vi "ESP301.vi"() -> ()   [LabVIEW 2014]
uses:
  ESP301/Newport ESP301.lvlib
panel:
  in  "stop":bool
  in  "AxisNumTiltY":dbl
  in  "AxisNumTiltX":dbl
  in  "AxisNumZ":dbl
  in  "AxisNumY":dbl
  in  "AxisNumX":dbl
  in  "Tilt  Y":T1 {"Actual Velocity" min=0.0 max=12.7 format="%1.5g"; "Move Relative" min=0.0 max=12.0 format="%1.5f"; "Set Velocity" min=0.0 max=0.2 format="%1.4f"; "Actual Position" format="%1.6f"; "Move Absolute" min=0.0 max=12.7 format="%1.5f"}
  in  "Tilt  X":T1 {"Actual Velocity" min=0.0 max=12.7 format="%1.5g"; "Move Relative" min=0.0 max=12.0 format="%1.5f"; "Set Velocity" min=0.0 max=0.2 format="%1.4f"; "Actual Position" format="%1.6f"; "Move Absolute" min=0.0 max=12.7 format="%1.5f"}
  in  "Axis Z":T1 {"Actual Velocity" min=0.0 max=12.7 format="%1.5g"; "Move Relative" min=0.0 max=12.0 format="%1.5f"; "Set Velocity" min=0.0 max=0.2 format="%1.4f"; "Actual Position" format="%1.6f"; "Move Absolute" min=0.0 max=12.7 format="%1.5f"}
  in  "Axis Y":T1 {"Actual Velocity" min=0.0 max=12.7 format="%1.5g"; "Move Relative" min=0.0 max=12.0 format="%1.5f"; "Set Velocity" min=0.0 max=0.2 format="%1.4f"; "Actual Position" format="%1.6f"; "Move Absolute" min=0.0 max=12.7 format="%1.5f"}
  in  "Axis X":T1 {"Actual Velocity" min=0.0 max=12.7 format="%1.5g"; "Move Relative" min=0.0 max=12.0 format="%1.5f"; "Set Velocity" min=0.0 max=0.2 format="%1.4f"; "Actual Position" format="%1.6f"; "Move Absolute" min=0.0 max=12.7 format="%1.5f"}
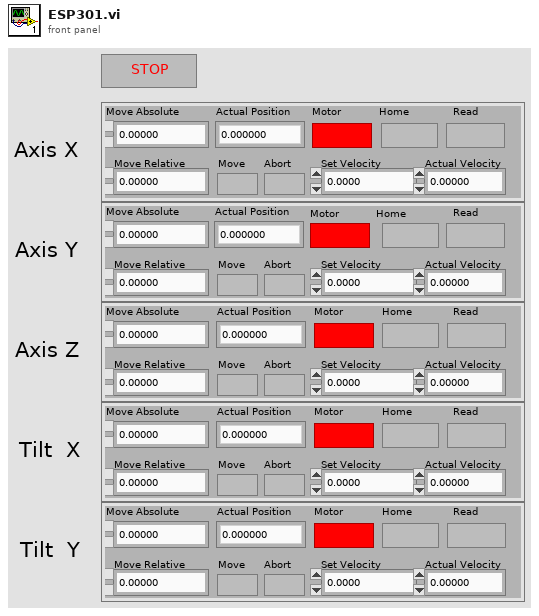
[diagram p1: front panel]
types:
  T1 = cluster{"Move Absolute":dbl, "Actual Position":dbl, "Motor":bool, "Home":bool, "Set Velocity":dbl, "Move Relative":dbl, "Actual Velocity":dbl, "Move":bool, "Read":bool, "Abort":bool}
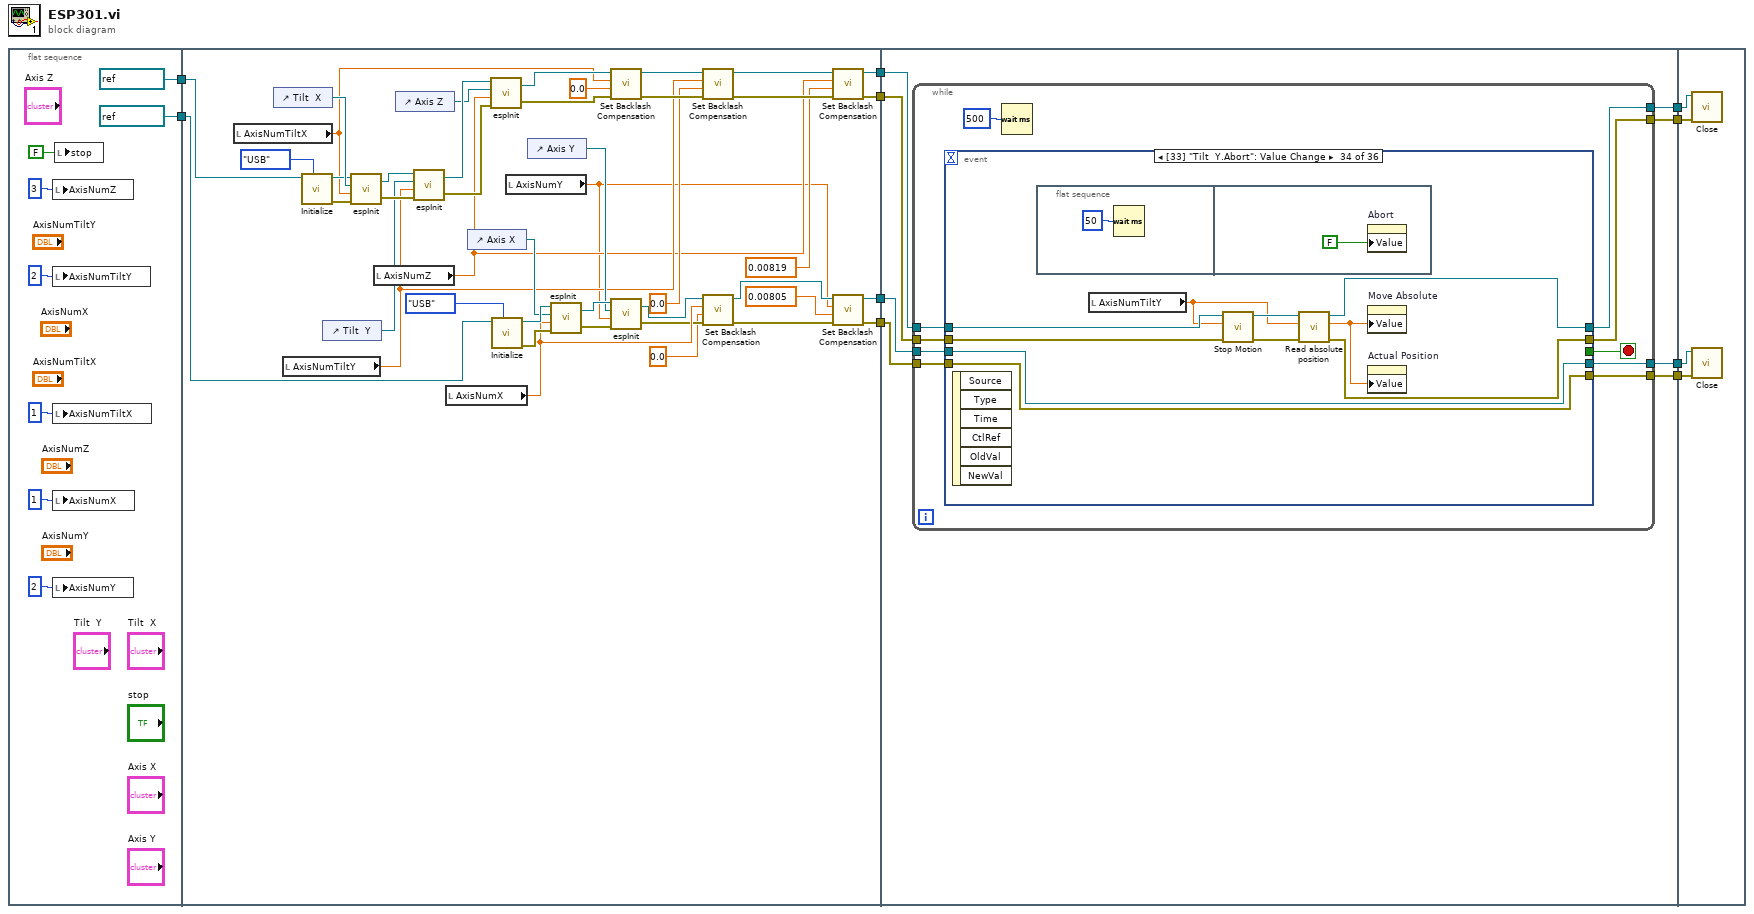
[diagram p0: block diagram]
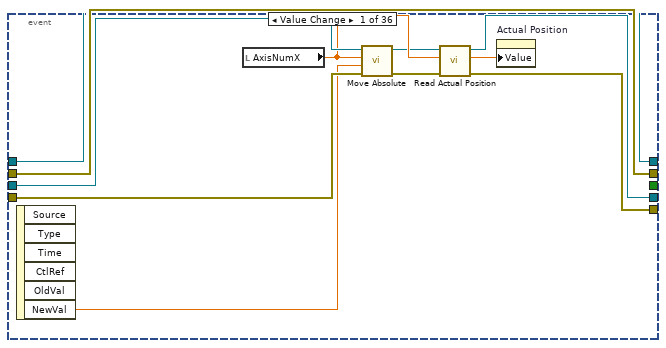
[diagram p2: hidden frame]
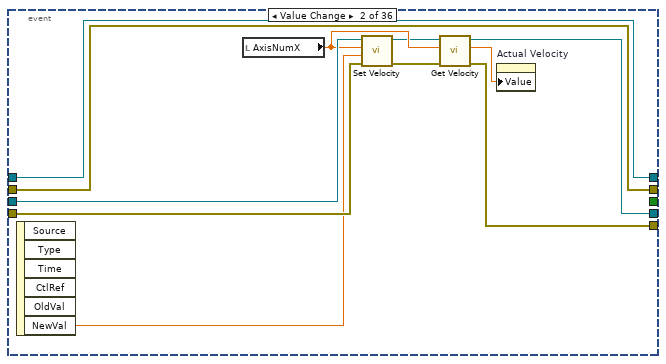
[diagram p3: hidden frame]
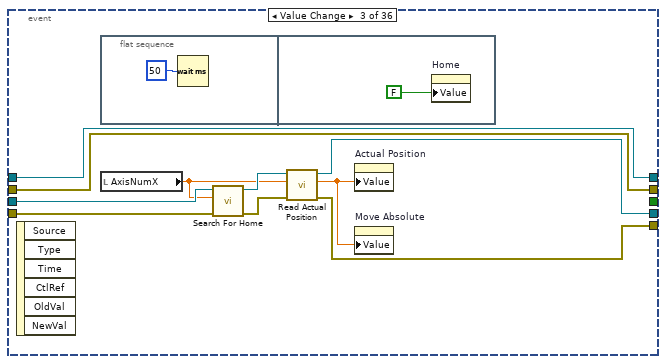
[diagram p4: hidden frame]
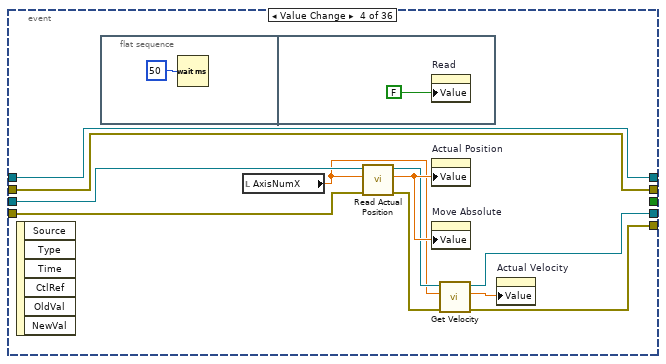
[diagram p5: hidden frame]
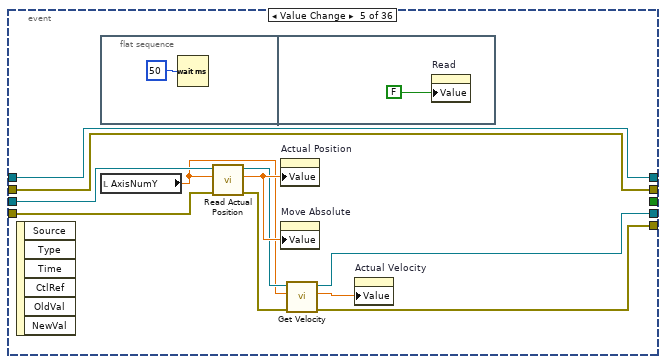
[diagram p6: hidden frame]
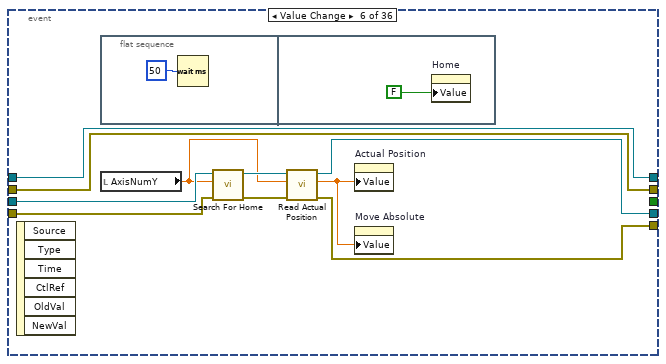
[diagram p7: hidden frame]
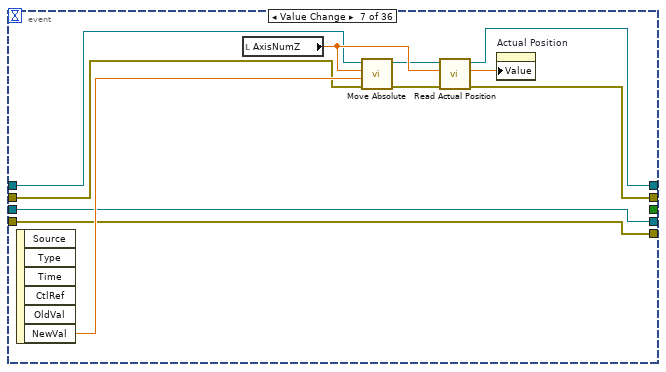
[diagram p8: hidden frame]
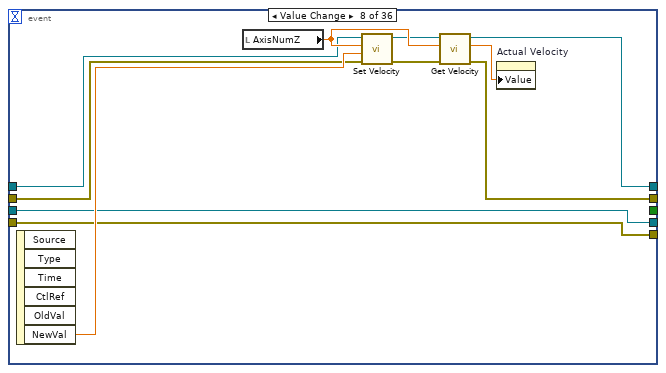
[diagram p9: hidden frame]
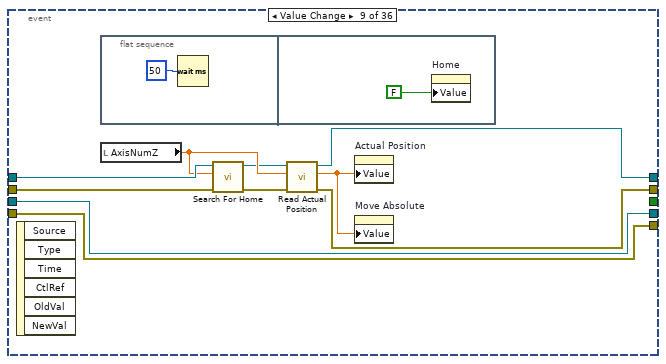
[diagram p10: hidden frame]
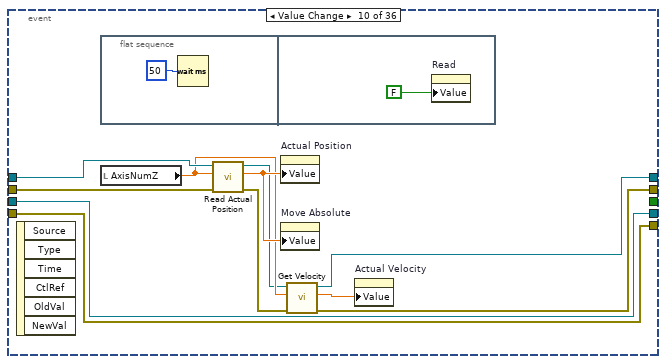
[diagram p11: hidden frame]
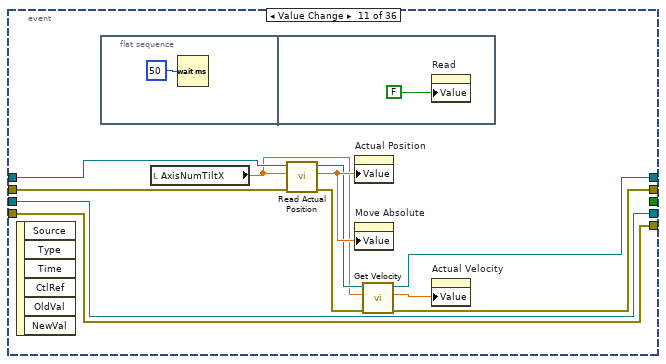
[diagram p12: hidden frame]
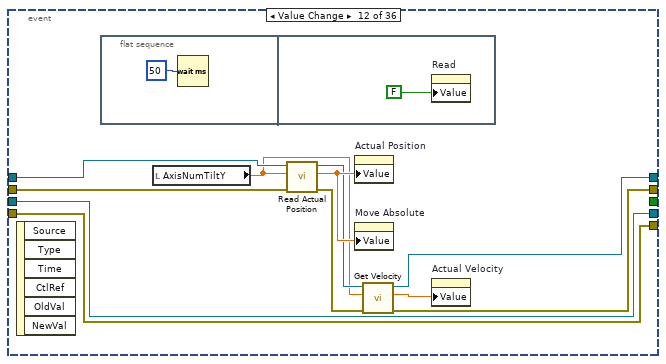
[diagram p13: hidden frame]
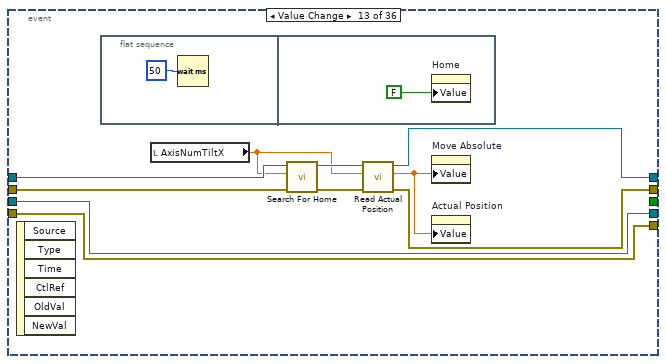
[diagram p14: hidden frame]
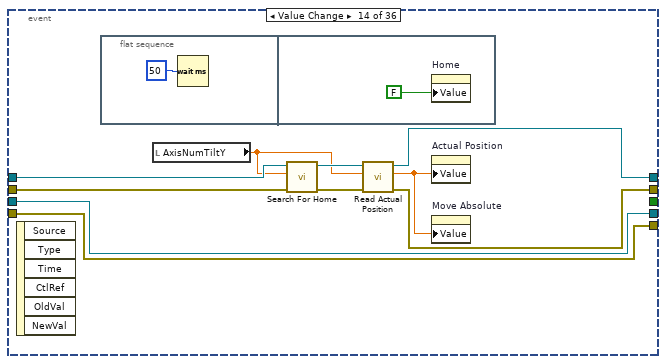
[diagram p15: hidden frame]
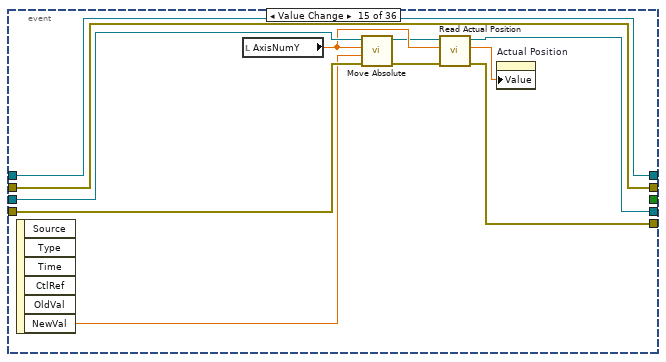
[diagram p16: hidden frame]
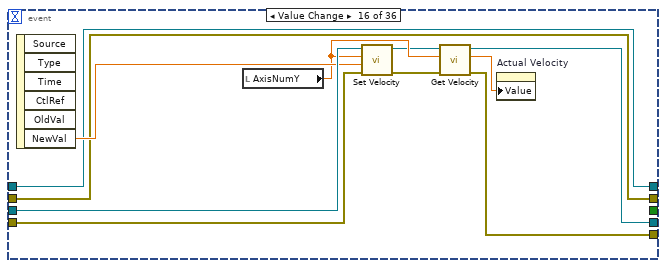
[diagram p17: hidden frame]
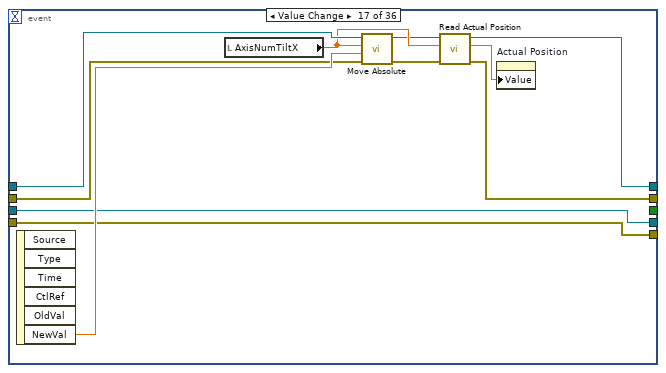
[diagram p18: hidden frame]
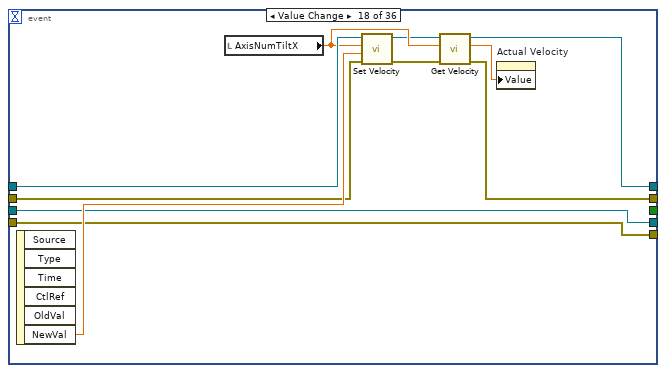
[diagram p19: hidden frame]
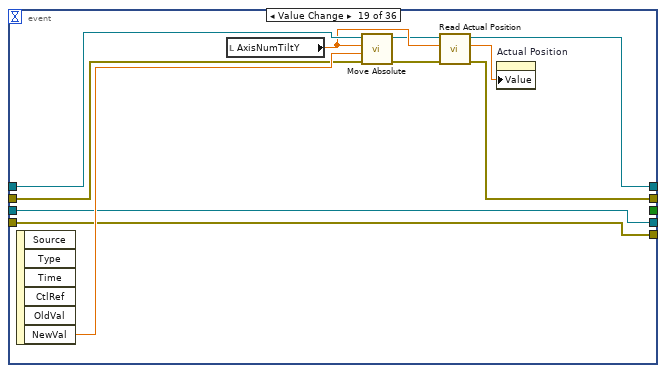
[diagram p20: hidden frame]
diagram:
  n1 = flat-sequence {
    tunnel: [refnum<visa-resource-name> "COM4" ("VISA resource name")] -> w7
    tunnel: [refnum<visa-resource-name> "COM5" ("VISA resource name")] -> w6
    tunnel: [w23] -> w10
    tunnel: [w30] -> w9
    tunnel: [w29] -> w8
    tunnel: w7 -> [w44]
    tunnel: w6 -> [w43]
    tunnel: [w24] -> w5
    tunnel: w10 -> [w68]
    tunnel: w9 -> [w67]
    tunnel: w8 -> [w66]
    tunnel: w5 -> [w69]
    tunnel: [w65] -> w4
    tunnel: [w64] -> w3
    tunnel: [w63] -> w2
    tunnel: [w62] -> w1
    tunnel: w4 -> [w489]
    tunnel: w3 -> [w492]
    tunnel: w2 -> [w491]
    tunnel: w1 -> [w490]
    frame #0 {
      n2 = local write "AxisNumZ"(3) -> ()
      n3 = local write "AxisNumTiltY"(2) -> ()
      n4 = local write "AxisNumTiltX"(1) -> ()
      n5 = local write "AxisNumX"(1 ("AxisNumX")) -> ()
      n6 = local write "AxisNumY"(2) -> ()
      n7 = local write "stop"(FALSE) -> ()
    }
    frame #1 {
      n8 = local read "AxisNumTiltX"() -> (w39:dbl)
      n9 = control-ref of="Tilt  X"() -> (w50:refnum<vi>)
      n10 = local read "AxisNumTiltY"() -> (w36:dbl)
      n11 = call <instrlib>:"Initialize.vi"("VISA resource name"=w44, "Serial Link (RS232)"=enum16{"RS232", "USB"}."USB") -> ("VISA resource name out"=w49:refnum<visa-resource-name>, "error out"=w58:errorcluster)  [unwired: 7 in]
      n12 = control-ref of="Tilt  Y"() -> (w47:refnum<vi>)
      n13 = call "espInit.vi"("error in (no error)"=w58, "Axis"=w39, "RefNum"=w50, "VISA resource name in"=w49) -> ("error out"=w56:errorcluster, "VISA resource name out"=w57:refnum<visa-resource-name>)
      n14 = local read "AxisNumZ"() -> (w32:dbl)
      n15 = control-ref of="Axis Z"() -> (w48:refnum<vi>)
      n16 = call "espInit.vi"("error in (no error)"=w56, "Axis"=w36, "RefNum"=w47, "VISA resource name in"=w57) -> ("error out"=w54:errorcluster, "VISA resource name out"=w55:refnum<visa-resource-name>)
      n17 = local read "AxisNumX"() -> (w26:dbl)
      n18 = control-ref of="Axis X"() -> (w46:refnum<vi>)
      n19 = call "espInit.vi"("error in (no error)"=w54, "Axis"=w32, "RefNum"=w48, "VISA resource name in"=w55) -> ("error out"=w41:errorcluster, "VISA resource name out"=w42:refnum<visa-resource-name>)
      n20 = call <instrlib>:"Initialize.vi"("VISA resource name"=w43, "Serial Link (RS232)"=enum16{"RS232", "USB"}."USB") -> ("VISA resource name out"=w52:refnum<visa-resource-name>, "error out"=w51:errorcluster)  [unwired: 7 in]
      n21 = local read "AxisNumY"() -> (w25:dbl)
      n22 = control-ref of="Axis Y"() -> (w45:refnum<vi>)
      n23 = call "espInit.vi"("error in (no error)"=w51, "Axis"=w26, "RefNum"=w46, "VISA resource name in"=w52) -> ("error out"=w60:errorcluster, "VISA resource name out"=w61:refnum<visa-resource-name>)
      n24 = call <instrlib>:"Set Backlash Compensation.vi"("error in (no error)"=w41, "Backlash Compensation Value (0 units)"=0.0, "Axis (1)"=w39, "VISA resource name"=w42) -> ("error out"=w37:errorcluster, "VISA resource name out"=w38:refnum<visa-resource-name>)  [unwired: 2 in]
      n25 = call "espInit.vi"("error in (no error)"=w60, "Axis"=w25, "RefNum"=w45, "VISA resource name in"=w61) -> ("error out"=w21:errorcluster, "VISA resource name out"=w22:refnum<visa-resource-name>)
      n26 = call <instrlib>:"Set Backlash Compensation.vi"("error in (no error)"=w37, "Backlash Compensation Value (0 units)"=0.0, "Axis (1)"=w36, "VISA resource name"=w38) -> ("error out"=w33:errorcluster, "VISA resource name out"=w34:refnum<visa-resource-name>)  [unwired: 2 in]
      n27 = call <instrlib>:"Set Backlash Compensation.vi"("error in (no error)"=w21, "Backlash Compensation Value (0 units)"=0.0, "Axis (1)"=w26, "VISA resource name"=w22) -> ("error out"=w27:errorcluster, "VISA resource name out"=w28:refnum<visa-resource-name>)  [unwired: 2 in]
      n28 = call <instrlib>:"Set Backlash Compensation.vi"("error in (no error)"=w33, "Backlash Compensation Value (0 units)"=0.00819, "Axis (1)"=w32, "VISA resource name"=w34) -> ("error out"=w29:errorcluster, "VISA resource name out"=w30:refnum<visa-resource-name>)  [unwired: 2 in]
      n29 = call <instrlib>:"Set Backlash Compensation.vi"("error in (no error)"=w27, "Backlash Compensation Value (0 units)"=0.00805, "Axis (1)"=w25, "VISA resource name"=w28) -> ("error out"=w23:errorcluster, "VISA resource name out"=w24:refnum<visa-resource-name>)  [unwired: 2 in]
    }
    frame #2 {
      n30 = while {
        tunnel: w67 -> [w79]
        tunnel: w66 -> [w78]
        tunnel: w69 -> [w77]
        tunnel: w68 -> [w76]
        tunnel: [w75] -> w65
        tunnel: [w74] -> w64
        tunnel: [w73] -> w63
        tunnel: [w72] -> w62
        stop <- w70 stop-if-true
        n31 = event shown="[33] \"Tilt  Y.Abort\": Value Change" {
          selector: _ -> [_ _ _ _ _ _ _ _ _ _ _ _ _ _ _ _ _ _ _ _ _ _ _ _ _ _ _ _ _ _ _ _ _ _ _ _]
          dyn-events: _ -> [_ _ _ _ _ _ _ _ _ _ _ _ _ _ _ _ _ _ _ _ _ _ _ _ _ _ _ _ _ _ _ _ _ _ _ _]
          timeout: _ -> [_ _ _ _ _ _ _ _ _ _ _ _ _ _ _ _ _ _ _ _ _ _ _ _ _ _ _ _ _ _ _ _ _ _ _ _]
          tunnel: w79 -> [w81 w92 w103 w121 w134 w141 w157 w168 w183 w195 w209 w222 w234 w246 w252 w263 w279 w290 w301 w312 w316 w330 w340 w347 w359 w363 w375 w383 w387 w405 w419 w433 w451 w463 _ w478]
          tunnel: w78 -> [w80 w91 w102 w120 w133 w140 w156 w167 w182 w194 w208 w221 w233 w245 w251 w262 w278 w289 w300 w311 w315 w329 w341 w346 w358 w362 w374 w382 w386 w404 w418 w432 w450 w462 w466 w477]
          tunnel: w77 -> [w90 w101 w111 w124 w137 w149 w153 w164 w175 w193 w206 w219 w225 w238 w259 w270 w274 w285 w296 w307 w325 w334 w339 w344 w351 w367 w370 w381 w396 w401 w414 w429 w443 w455 w470 w482]
          tunnel: w76 -> [w89 w100 w110 w123 w136 w148 w152 w163 w174 w192 w205 w218 w226 w237 w258 w269 w273 w284 w295 w306 w324 w333 w338 w342 w350 w366 w373 w380 w395 w400 w415 w428 w442 w454 w469 w481]
          tunnel: [w87 w98 w107 w116 w130 w143 w153 w164 w175 w193 w206 w219 w225 w238 w255 w266 w274 w285 w296 w307 w320 w332 w339 w344 w351 w365 w370 w381 w391 w401 w414 w429 w443 w455 w468 w480] -> w73
          tunnel: [w86 w97 w106 w115 w129 w147 w152 w163 w174 w192 w205 w218 w226 w237 w254 w265 w273 w284 w295 w306 w319 w331 w338 w342 w350 w364 w373 w380 w390 w400 w415 w428 w442 w454 w467 w479] -> w72
          tunnel: [w81 w92 w103 w121 w134 w141 w160 w171 w181 w187 w199 w214 w232 w242 w252 w263 w276 w287 w298 w309 w316 w330 w340 w345 w355 w363 w371 w379 w387 w402 w416 w430 w447 w459 _ w478] -> w75
          tunnel: [w80 w91 w102 w120 w133 w140 w159 w170 w180 w186 w200 w213 w231 w241 w251 w262 w275 w286 w297 w308 w315 w329 w341 w343 w354 w362 w372 w378 w386 w403 w417 w431 w446 w458 w466 w477] -> w74
          tunnel: [_ _ _ _ _ _ _ _ _ _ _ _ _ _ _ _ _ _ _ _ _ _ w337 _ _ _ _ _ _ _ _ _ _ _ _ _] -> w70
          event "Axis X.Move Absolute": Value Change {
            n32 = event-data() -> ("NewVal"=w88:dbl)  [unwired: 1 in, 5 out]
            n33 = local read "AxisNumX"() -> (w84:dbl)
            n34 = call <instrlib>:"Move Absolute.vi"("error in (no error)"=w89, "Position (0 units)"=w88, "Axis (1)"=w84, "VISA resource name"=w90) -> ("error out"=w82:errorcluster, "VISA resource name out"=w83:refnum<visa-resource-name>)  [unwired: 2 in]
            n35 = call <instrlib>:"Read Actual Position.vi"("error in (no error)"=w82, "Axis (1)"=w84, "VISA resource name"=w83) -> ("error out"=w86:errorcluster, "Position (units)"=w85:dbl, "VISA resource name out"=w87:refnum<visa-resource-name>)  [unwired: 2 in]
            n36 = property on="Actual Position" class="DigNum (strict)"("Value"=w85) -> ()  [unwired: 2 in, 2 out]
          }
          event "Axis X.Set Velocity": Value Change {
            n37 = event-data() -> ("NewVal"=w99:dbl)  [unwired: 1 in, 5 out]
            n38 = local read "AxisNumX"() -> (w95:dbl)
            n39 = call <instrlib>:"Set Velocity.vi"("error in (no error)"=w100, "Velocity (units/s)"=w99, "Axis (1)"=w95, "VISA resource name"=w101) -> ("error out"=w93:errorcluster, "VISA resource name out"=w94:refnum<visa-resource-name>)  [unwired: 2 in]
            n40 = call "Get Velocity.vi"("error in (no error)"=w93, "Axis (1)"=w95, "VISA resource name"=w94) -> ("error out"=w97:errorcluster, "Velocity (units/s)"=w96:dbl, "VISA resource name out"=w98:refnum<visa-resource-name>)  [unwired: 2 in]
            n41 = property on="Actual Velocity" class="DigNum (strict)"("Value"=w96) -> ()  [unwired: 2 in, 2 out]
          }
          event "Axis X.Home": Value Change {
            n42 = event-data() -> ()  [unwired: 1 in, 6 out]
            n43 = flat-sequence {
              frame #0 {
                n44 = Wait (ms)(milliseconds to wait=u32 50) -> ()  [unwired: 1 out]
              }
              frame #1 {
                n45 = property on="Home" class="Bool (strict)"("Value"=FALSE) -> ()  [unwired: 2 in, 2 out]
              }
            }
            n46 = local read "AxisNumX"() -> (w105:dbl)
            n47 = call <instrlib>:"Search For Home.vi"("error in (no error)"=w110, "Axis (1)"=w105, "VISA resource name"=w111) -> ("error out"=w108:errorcluster, "VISA resource name out"=w109:refnum<visa-resource-name>)  [unwired: 4 in]
            n48 = call <instrlib>:"Read Actual Position.vi"("error in (no error)"=w108, "Axis (1)"=w105, "VISA resource name"=w109) -> ("error out"=w106:errorcluster, "Position (units)"=w104:dbl, "VISA resource name out"=w107:refnum<visa-resource-name>)  [unwired: 2 in]
            n49 = property on="Actual Position" class="DigNum (strict)"("Value"=w104) -> ()  [unwired: 2 in, 2 out]
            n50 = property on="Move Absolute" class="DigNum (strict)"("Value"=w104) -> ()  [unwired: 2 in, 2 out]
          }
          event "Axis X.Read": Value Change {
            n51 = event-data() -> ()  [unwired: 1 in, 6 out]
            n52 = flat-sequence {
              frame #0 {
                n53 = Wait (ms)(milliseconds to wait=u32 50) -> ()  [unwired: 1 out]
              }
              frame #1 {
                n54 = property on="Read" class="Bool (strict)"("Value"=FALSE) -> ()  [unwired: 2 in, 2 out]
              }
            }
            n55 = local read "AxisNumX"() -> (w117:dbl)
            n56 = call <instrlib>:"Read Actual Position.vi"("error in (no error)"=w123, "Axis (1)"=w117, "VISA resource name"=w124) -> ("error out"=w118:errorcluster, "Position (units)"=w122:dbl, "VISA resource name out"=w119:refnum<visa-resource-name>)  [unwired: 2 in]
            n57 = property on="Actual Position" class="DigNum (strict)"("Value"=w122) -> ()  [unwired: 2 in, 2 out]
            n58 = property on="Move Absolute" class="DigNum (strict)"("Value"=w122) -> ()  [unwired: 2 in, 2 out]
            n59 = call "Get Velocity.vi"("error in (no error)"=w118, "Axis (1)"=w117, "VISA resource name"=w119) -> ("error out"=w115:errorcluster, "Velocity (units/s)"=w114:dbl, "VISA resource name out"=w116:refnum<visa-resource-name>)  [unwired: 2 in]
            n60 = property on="Actual Velocity" class="DigNum (strict)"("Value"=w114) -> ()  [unwired: 2 in, 2 out]
          }
          event "Axis Y.Read": Value Change {
            n61 = event-data() -> ()  [unwired: 1 in, 6 out]
            n62 = flat-sequence {
              frame #0 {
                n63 = Wait (ms)(milliseconds to wait=u32 50) -> ()  [unwired: 1 out]
              }
              frame #1 {
                n64 = property on="Read" class="Bool (strict)"("Value"=FALSE) -> ()  [unwired: 2 in, 2 out]
              }
            }
            n65 = local read "AxisNumY"() -> (w128:dbl)
            n66 = call <instrlib>:"Read Actual Position.vi"("error in (no error)"=w136, "Axis (1)"=w128, "VISA resource name"=w137) -> ("error out"=w131:errorcluster, "Position (units)"=w135:dbl, "VISA resource name out"=w132:refnum<visa-resource-name>)  [unwired: 2 in]
            n67 = property on="Actual Position" class="DigNum (strict)"("Value"=w135) -> ()  [unwired: 2 in, 2 out]
            n68 = property on="Move Absolute" class="DigNum (strict)"("Value"=w135) -> ()  [unwired: 2 in, 2 out]
            n69 = call "Get Velocity.vi"("error in (no error)"=w131, "Axis (1)"=w128, "VISA resource name"=w132) -> ("error out"=w129:errorcluster, "Velocity (units/s)"=w127:dbl, "VISA resource name out"=w130:refnum<visa-resource-name>)  [unwired: 2 in]
            n70 = property on="Actual Velocity" class="DigNum (strict)"("Value"=w127) -> ()  [unwired: 2 in, 2 out]
          }
          event "Axis Y.Home": Value Change {
            n71 = event-data() -> ()  [unwired: 1 in, 6 out]
            n72 = flat-sequence {
              frame #0 {
                n73 = Wait (ms)(milliseconds to wait=u32 50) -> ()  [unwired: 1 out]
              }
              frame #1 {
                n74 = property on="Home" class="Bool (strict)"("Value"=FALSE) -> ()  [unwired: 2 in, 2 out]
              }
            }
            n75 = local read "AxisNumY"() -> (w144:dbl)
            n76 = call <instrlib>:"Search For Home.vi"("error in (no error)"=w148, "Axis (1)"=w144, "VISA resource name"=w149) -> ("error out"=w145:errorcluster, "VISA resource name out"=w146:refnum<visa-resource-name>)  [unwired: 4 in]
            n77 = call <instrlib>:"Read Actual Position.vi"("error in (no error)"=w145, "Axis (1)"=w144, "VISA resource name"=w146) -> ("error out"=w147:errorcluster, "Position (units)"=w142:dbl, "VISA resource name out"=w143:refnum<visa-resource-name>)  [unwired: 2 in]
            n78 = property on="Actual Position" class="DigNum (strict)"("Value"=w142) -> ()  [unwired: 2 in, 2 out]
            n79 = property on="Move Absolute" class="DigNum (strict)"("Value"=w142) -> ()  [unwired: 2 in, 2 out]
          }
          event "Axis Z.Move Absolute": Value Change {
            n80 = event-data() -> ("NewVal"=w162:dbl)  [unwired: 1 in, 5 out]
            n81 = local read "AxisNumZ"() -> (w158:dbl)
            n82 = call <instrlib>:"Move Absolute.vi"("error in (no error)"=w156, "Position (0 units)"=w162, "Axis (1)"=w158, "VISA resource name"=w157) -> ("error out"=w154:errorcluster, "VISA resource name out"=w155:refnum<visa-resource-name>)  [unwired: 2 in]
            n83 = call <instrlib>:"Read Actual Position.vi"("error in (no error)"=w154, "Axis (1)"=w158, "VISA resource name"=w155) -> ("error out"=w159:errorcluster, "Position (units)"=w161:dbl, "VISA resource name out"=w160:refnum<visa-resource-name>)  [unwired: 2 in]
            n84 = property on="Actual Position" class="DigNum (strict)"("Value"=w161) -> ()  [unwired: 2 in, 2 out]
          }
          event "Axis Z.Set Velocity": Value Change {
            n85 = event-data() -> ("NewVal"=w173:dbl)  [unwired: 1 in, 5 out]
            n86 = local read "AxisNumZ"() -> (w169:dbl)
            n87 = call <instrlib>:"Set Velocity.vi"("error in (no error)"=w167, "Velocity (units/s)"=w173, "Axis (1)"=w169, "VISA resource name"=w168) -> ("error out"=w165:errorcluster, "VISA resource name out"=w166:refnum<visa-resource-name>)  [unwired: 2 in]
            n88 = call "Get Velocity.vi"("error in (no error)"=w165, "Axis (1)"=w169, "VISA resource name"=w166) -> ("error out"=w170:errorcluster, "Velocity (units/s)"=w172:dbl, "VISA resource name out"=w171:refnum<visa-resource-name>)  [unwired: 2 in]
            n89 = property on="Actual Velocity" class="DigNum (strict)"("Value"=w172) -> ()  [unwired: 2 in, 2 out]
          }
          event "Axis Z.Home": Value Change {
            n90 = event-data() -> ()  [unwired: 1 in, 6 out]
            n91 = flat-sequence {
              frame #0 {
                n92 = Wait (ms)(milliseconds to wait=u32 50) -> ()  [unwired: 1 out]
              }
              frame #1 {
                n93 = property on="Home" class="Bool (strict)"("Value"=FALSE) -> ()  [unwired: 2 in, 2 out]
              }
            }
            n94 = local read "AxisNumZ"() -> (w179:dbl)
            n95 = call <instrlib>:"Search For Home.vi"("error in (no error)"=w182, "Axis (1)"=w179, "VISA resource name"=w183) -> ("error out"=w178:errorcluster, "VISA resource name out"=w177:refnum<visa-resource-name>)  [unwired: 4 in]
            n96 = call <instrlib>:"Read Actual Position.vi"("error in (no error)"=w178, "Axis (1)"=w179, "VISA resource name"=w177) -> ("error out"=w180:errorcluster, "Position (units)"=w176:dbl, "VISA resource name out"=w181:refnum<visa-resource-name>)  [unwired: 2 in]
            n97 = property on="Actual Position" class="DigNum (strict)"("Value"=w176) -> ()  [unwired: 2 in, 2 out]
            n98 = property on="Move Absolute" class="DigNum (strict)"("Value"=w176) -> ()  [unwired: 2 in, 2 out]
          }
          event "Axis Z.Read": Value Change {
            n99 = event-data() -> ()  [unwired: 1 in, 6 out]
            n100 = flat-sequence {
              frame #0 {
                n101 = Wait (ms)(milliseconds to wait=u32 50) -> ()  [unwired: 1 out]
              }
              frame #1 {
                n102 = property on="Read" class="Bool (strict)"("Value"=FALSE) -> ()  [unwired: 2 in, 2 out]
              }
            }
            n103 = local read "AxisNumZ"() -> (w190:dbl)
            n104 = call <instrlib>:"Read Actual Position.vi"("error in (no error)"=w194, "Axis (1)"=w190, "VISA resource name"=w195) -> ("error out"=w188:errorcluster, "Position (units)"=w196:dbl, "VISA resource name out"=w189:refnum<visa-resource-name>)  [unwired: 2 in]
            n105 = property on="Actual Position" class="DigNum (strict)"("Value"=w196) -> ()  [unwired: 2 in, 2 out]
            n106 = property on="Move Absolute" class="DigNum (strict)"("Value"=w196) -> ()  [unwired: 2 in, 2 out]
            n107 = call "Get Velocity.vi"("error in (no error)"=w188, "Axis (1)"=w190, "VISA resource name"=w189) -> ("error out"=w186:errorcluster, "Velocity (units/s)"=w191:dbl, "VISA resource name out"=w187:refnum<visa-resource-name>)  [unwired: 2 in]
            n108 = property on="Actual Velocity" class="DigNum (strict)"("Value"=w191) -> ()  [unwired: 2 in, 2 out]
          }
          event "Tilt  X.Read": Value Change {
            n109 = event-data() -> ()  [unwired: 1 in, 6 out]
            n110 = flat-sequence {
              frame #0 {
                n111 = Wait (ms)(milliseconds to wait=u32 50) -> ()  [unwired: 1 out]
              }
              frame #1 {
                n112 = property on="Read" class="Bool (strict)"("Value"=FALSE) -> ()  [unwired: 2 in, 2 out]
              }
            }
            n113 = local read "AxisNumTiltX"() -> (w202:dbl)
            n114 = call <instrlib>:"Read Actual Position.vi"("error in (no error)"=w208, "Axis (1)"=w202, "VISA resource name"=w209) -> ("error out"=w201:errorcluster, "Position (units)"=w207:dbl, "VISA resource name out"=w203:refnum<visa-resource-name>)  [unwired: 2 in]
            n115 = property on="Actual Position" class="DigNum (strict)"("Value"=w207) -> ()  [unwired: 2 in, 2 out]
            n116 = property on="Move Absolute" class="DigNum (strict)"("Value"=w207) -> ()  [unwired: 2 in, 2 out]
            n117 = call "Get Velocity.vi"("error in (no error)"=w201, "Axis (1)"=w202, "VISA resource name"=w203) -> ("error out"=w200:errorcluster, "Velocity (units/s)"=w204:dbl, "VISA resource name out"=w199:refnum<visa-resource-name>)  [unwired: 2 in]
            n118 = property on="Actual Velocity" class="DigNum (strict)"("Value"=w204) -> ()  [unwired: 2 in, 2 out]
          }
          event "Tilt  Y.Read": Value Change {
            n119 = event-data() -> ()  [unwired: 1 in, 6 out]
            n120 = flat-sequence {
              frame #0 {
                n121 = Wait (ms)(milliseconds to wait=u32 50) -> ()  [unwired: 1 out]
              }
              frame #1 {
                n122 = property on="Read" class="Bool (strict)"("Value"=FALSE) -> ()  [unwired: 2 in, 2 out]
              }
            }
            n123 = local read "AxisNumTiltY"() -> (w212:dbl)
            n124 = call <instrlib>:"Read Actual Position.vi"("error in (no error)"=w221, "Axis (1)"=w212, "VISA resource name"=w222) -> ("error out"=w215:errorcluster, "Position (units)"=w220:dbl, "VISA resource name out"=w216:refnum<visa-resource-name>)  [unwired: 2 in]
            n125 = property on="Actual Position" class="DigNum (strict)"("Value"=w220) -> ()  [unwired: 2 in, 2 out]
            n126 = property on="Move Absolute" class="DigNum (strict)"("Value"=w220) -> ()  [unwired: 2 in, 2 out]
            n127 = call "Get Velocity.vi"("error in (no error)"=w215, "Axis (1)"=w212, "VISA resource name"=w216) -> ("error out"=w213:errorcluster, "Velocity (units/s)"=w217:dbl, "VISA resource name out"=w214:refnum<visa-resource-name>)  [unwired: 2 in]
            n128 = property on="Actual Velocity" class="DigNum (strict)"("Value"=w217) -> ()  [unwired: 2 in, 2 out]
          }
          event "Tilt  X.Home": Value Change {
            n129 = event-data() -> ()  [unwired: 1 in, 6 out]
            n130 = flat-sequence {
              frame #0 {
                n131 = Wait (ms)(milliseconds to wait=u32 50) -> ()  [unwired: 1 out]
              }
              frame #1 {
                n132 = property on="Home" class="Bool (strict)"("Value"=FALSE) -> ()  [unwired: 2 in, 2 out]
              }
            }
            n133 = local read "AxisNumTiltX"() -> (w228:dbl)
            n134 = call <instrlib>:"Search For Home.vi"("error in (no error)"=w233, "Axis (1)"=w228, "VISA resource name"=w234) -> ("error out"=w230:errorcluster, "VISA resource name out"=w229:refnum<visa-resource-name>)  [unwired: 4 in]
            n135 = call <instrlib>:"Read Actual Position.vi"("error in (no error)"=w230, "Axis (1)"=w228, "VISA resource name"=w229) -> ("error out"=w231:errorcluster, "Position (units)"=w227:dbl, "VISA resource name out"=w232:refnum<visa-resource-name>)  [unwired: 2 in]
            n136 = property on="Move Absolute" class="DigNum (strict)"("Value"=w227) -> ()  [unwired: 2 in, 2 out]
            n137 = property on="Actual Position" class="DigNum (strict)"("Value"=w227) -> ()  [unwired: 2 in, 2 out]
          }
          event "Tilt  Y.Home": Value Change {
            n138 = event-data() -> ()  [unwired: 1 in, 6 out]
            n139 = flat-sequence {
              frame #0 {
                n140 = Wait (ms)(milliseconds to wait=u32 50) -> ()  [unwired: 1 out]
              }
              frame #1 {
                n141 = property on="Home" class="Bool (strict)"("Value"=FALSE) -> ()  [unwired: 2 in, 2 out]
              }
            }
            n142 = local read "AxisNumTiltY"() -> (w240:dbl)
            n143 = call <instrlib>:"Search For Home.vi"("error in (no error)"=w245, "Axis (1)"=w240, "VISA resource name"=w246) -> ("error out"=w243:errorcluster, "VISA resource name out"=w244:refnum<visa-resource-name>)  [unwired: 4 in]
            n144 = call <instrlib>:"Read Actual Position.vi"("error in (no error)"=w243, "Axis (1)"=w240, "VISA resource name"=w244) -> ("error out"=w241:errorcluster, "Position (units)"=w239:dbl, "VISA resource name out"=w242:refnum<visa-resource-name>)  [unwired: 2 in]
            n145 = property on="Actual Position" class="DigNum (strict)"("Value"=w239) -> ()  [unwired: 2 in, 2 out]
            n146 = property on="Move Absolute" class="DigNum (strict)"("Value"=w239) -> ()  [unwired: 2 in, 2 out]
          }
          event "Axis Y.Move Absolute": Value Change {
            n147 = event-data() -> ("NewVal"=w257:dbl)  [unwired: 1 in, 5 out]
            n148 = local read "AxisNumY"() -> (w253:dbl)
            n149 = call <instrlib>:"Move Absolute.vi"("error in (no error)"=w258, "Position (0 units)"=w257, "Axis (1)"=w253, "VISA resource name"=w259) -> ("error out"=w249:errorcluster, "VISA resource name out"=w250:refnum<visa-resource-name>)  [unwired: 2 in]
            n150 = call <instrlib>:"Read Actual Position.vi"("error in (no error)"=w249, "Axis (1)"=w253, "VISA resource name"=w250) -> ("error out"=w254:errorcluster, "Position (units)"=w256:dbl, "VISA resource name out"=w255:refnum<visa-resource-name>)  [unwired: 2 in]
            n151 = property on="Actual Position" class="DigNum (strict)"("Value"=w256) -> ()  [unwired: 2 in, 2 out]
          }
          event "Axis Y.Set Velocity": Value Change {
            n152 = event-data() -> ("NewVal"=w268:dbl)  [unwired: 1 in, 5 out]
            n153 = local read "AxisNumY"() -> (w264:dbl)
            n154 = call <instrlib>:"Set Velocity.vi"("error in (no error)"=w269, "Velocity (units/s)"=w268, "Axis (1)"=w264, "VISA resource name"=w270) -> ("error out"=w260:errorcluster, "VISA resource name out"=w261:refnum<visa-resource-name>)  [unwired: 2 in]
            n155 = call "Get Velocity.vi"("error in (no error)"=w260, "Axis (1)"=w264, "VISA resource name"=w261) -> ("error out"=w265:errorcluster, "Velocity (units/s)"=w267:dbl, "VISA resource name out"=w266:refnum<visa-resource-name>)  [unwired: 2 in]
            n156 = property on="Actual Velocity" class="DigNum (strict)"("Value"=w267) -> ()  [unwired: 2 in, 2 out]
          }
          event "Tilt  X.Move Absolute": Value Change {
            n157 = event-data() -> ("NewVal"=w281:dbl)  [unwired: 1 in, 5 out]
            n158 = local read "AxisNumTiltX"() -> (w277:dbl)
            n159 = call <instrlib>:"Move Absolute.vi"("error in (no error)"=w278, "Position (0 units)"=w281, "Axis (1)"=w277, "VISA resource name"=w279) -> ("error out"=w271:errorcluster, "VISA resource name out"=w272:refnum<visa-resource-name>)  [unwired: 2 in]
            n160 = call <instrlib>:"Read Actual Position.vi"("error in (no error)"=w271, "Axis (1)"=w277, "VISA resource name"=w272) -> ("error out"=w275:errorcluster, "Position (units)"=w280:dbl, "VISA resource name out"=w276:refnum<visa-resource-name>)  [unwired: 2 in]
            n161 = property on="Actual Position" class="DigNum (strict)"("Value"=w280) -> ()  [unwired: 2 in, 2 out]
          }
          event "Tilt  X.Set Velocity": Value Change {
            n162 = event-data() -> ("NewVal"=w292:dbl)  [unwired: 1 in, 5 out]
            n163 = local read "AxisNumTiltX"() -> (w288:dbl)
            n164 = call <instrlib>:"Set Velocity.vi"("error in (no error)"=w289, "Velocity (units/s)"=w292, "Axis (1)"=w288, "VISA resource name"=w290) -> ("error out"=w282:errorcluster, "VISA resource name out"=w283:refnum<visa-resource-name>)  [unwired: 2 in]
            n165 = call "Get Velocity.vi"("error in (no error)"=w282, "Axis (1)"=w288, "VISA resource name"=w283) -> ("error out"=w286:errorcluster, "Velocity (units/s)"=w291:dbl, "VISA resource name out"=w287:refnum<visa-resource-name>)  [unwired: 2 in]
            n166 = property on="Actual Velocity" class="DigNum (strict)"("Value"=w291) -> ()  [unwired: 2 in, 2 out]
          }
          event "Tilt  Y.Move Absolute": Value Change {
            n167 = event-data() -> ("NewVal"=w303:dbl)  [unwired: 1 in, 5 out]
            n168 = local read "AxisNumTiltY"() -> (w299:dbl)
            n169 = call <instrlib>:"Move Absolute.vi"("error in (no error)"=w300, "Position (0 units)"=w303, "Axis (1)"=w299, "VISA resource name"=w301) -> ("error out"=w293:errorcluster, "VISA resource name out"=w294:refnum<visa-resource-name>)  [unwired: 2 in]
            n170 = call <instrlib>:"Read Actual Position.vi"("error in (no error)"=w293, "Axis (1)"=w299, "VISA resource name"=w294) -> ("error out"=w297:errorcluster, "Position (units)"=w302:dbl, "VISA resource name out"=w298:refnum<visa-resource-name>)  [unwired: 2 in]
            n171 = property on="Actual Position" class="DigNum (strict)"("Value"=w302) -> ()  [unwired: 2 in, 2 out]
          }
          event "Tilt  Y.Set Velocity": Value Change {
            n172 = event-data() -> ("NewVal"=w314:dbl)  [unwired: 1 in, 5 out]
            n173 = local read "AxisNumTiltY"() -> (w310:dbl)
            n174 = call <instrlib>:"Set Velocity.vi"("error in (no error)"=w311, "Velocity (units/s)"=w314, "Axis (1)"=w310, "VISA resource name"=w312) -> ("error out"=w304:errorcluster, "VISA resource name out"=w305:refnum<visa-resource-name>)  [unwired: 2 in]
            n175 = call "Get Velocity.vi"("error in (no error)"=w304, "Axis (1)"=w310, "VISA resource name"=w305) -> ("error out"=w308:errorcluster, "Velocity (units/s)"=w313:dbl, "VISA resource name out"=w309:refnum<visa-resource-name>)  [unwired: 2 in]
            n176 = property on="Actual Velocity" class="DigNum (strict)"("Value"=w313) -> ()  [unwired: 2 in, 2 out]
          }
          event "Axis X.Move": Value Change {
            n177 = event-data() -> ()  [unwired: 1 in, 6 out]
            n178 = flat-sequence {
              frame #0 {
                n179 = Wait (ms)(milliseconds to wait=u32 50) -> ()  [unwired: 1 out]
                n180 = property on="Move Relative" class="DigNum (strict)"("Value"=0) -> ()  [unwired: 2 in, 2 out]
              }
              frame #1 {
                n181 = property on="Move" class="Bool (strict)"("Value"=FALSE) -> ()  [unwired: 2 in, 2 out]
              }
            }
            n182 = property on="Move Relative" class="DigNum (strict)"() -> ("Value"=w318:dbl)  [unwired: 2 in, 2 out]
            n183 = local read "AxisNumX"() -> (w321:dbl)
            n184 = call <instrlib>:"Move Relative.vi"("error in (no error)"=w324, "Position (0 units)"=w318, "Axis (1)"=w321, "VISA resource name"=w325) -> ("error out"=w322:errorcluster, "VISA resource name out"=w323:refnum<visa-resource-name>)  [unwired: 2 in]
            n185 = call <instrlib>:"Read Actual Position.vi"("error in (no error)"=w322, "Axis (1)"=w321, "VISA resource name"=w323) -> ("error out"=w319:errorcluster, "Position (units)"=w317:dbl, "VISA resource name out"=w320:refnum<visa-resource-name>)  [unwired: 2 in]
            n186 = property on="Move Absolute" class="DigNum (strict)"("Value"=w317) -> ()  [unwired: 2 in, 2 out]
            n187 = property on="Actual Position" class="DigNum (strict)"("Value"=w317) -> ()  [unwired: 2 in, 2 out]
          }
          event "Axis X.Motor": Value Change {
            n188 = event-data() -> ("NewVal"=w335:bool)  [unwired: 1 in, 5 out]
            n189 = local read "AxisNumX"() -> (w336:dbl)
            n190 = call <instrlib>:"Enable Disable Motor.vi"("error in (no error)"=w333, "Action (OFF)"=w335, "Axis (1)"=w336, "VISA resource name"=w334) -> ("error out"=w331:errorcluster, "VISA resource name out"=w332:refnum<visa-resource-name>)  [unwired: 2 in]
          }
          event "stop": Value Change {
            n191 = event-data() -> ("NewVal"=w337:bool)  [unwired: 1 in, 5 out]
          }
          event "Axis Z.Motor": Value Change {
            n192 = event-data() -> ("NewVal"=w348:bool)  [unwired: 1 in, 5 out]
            n193 = local read "AxisNumZ"() -> (w349:dbl)
            n194 = call <instrlib>:"Enable Disable Motor.vi"("error in (no error)"=w346, "Action (OFF)"=w348, "Axis (1)"=w349, "VISA resource name"=w347) -> ("error out"=w343:errorcluster, "VISA resource name out"=w345:refnum<visa-resource-name>)  [unwired: 2 in]
          }
          event "Axis Z.Abort": Value Change {
            n195 = event-data() -> ()  [unwired: 1 in, 6 out]
            n196 = flat-sequence {
              frame #0 {
                n197 = Wait (ms)(milliseconds to wait=u32 50) -> ()  [unwired: 1 out]
              }
              frame #1 {
                n198 = property on="Abort" class="Bool (strict)"("Value"=FALSE) -> ()  [unwired: 2 in, 2 out]
              }
            }
            n199 = local read "AxisNumZ"() -> (w353:dbl)
            n200 = call <instrlib>:"Stop Motion.vi"("error in (no error)"=w358, "Axis (1)"=w353, "VISA resource name"=w359) -> ("error out"=w356:errorcluster, "VISA resource name out"=w357:refnum<visa-resource-name>)  [unwired: 3 in]
            n201 = call <instrlib>:"Read absolute position.vi"("error in (no error)"=w356, "Axis (1)"=w353, "VISA resource name"=w357) -> ("error out"=w354:errorcluster, "Position (units)"=w352:dbl, "VISA resource name out"=w355:refnum<visa-resource-name>)  [unwired: 2 in]
            n202 = property on="Actual Position" class="DigNum (strict)"("Value"=w352) -> ()  [unwired: 2 in, 2 out]
            n203 = property on="Move Absolute" class="DigNum (strict)"("Value"=w352) -> ()  [unwired: 2 in, 2 out]
          }
          event "Axis Y.Motor": Value Change {
            n204 = event-data() -> ("NewVal"=w368:bool)  [unwired: 1 in, 5 out]
            n205 = local read "AxisNumY"() -> (w369:dbl)
            n206 = call <instrlib>:"Enable Disable Motor.vi"("error in (no error)"=w366, "Action (OFF)"=w368, "Axis (1)"=w369, "VISA resource name"=w367) -> ("error out"=w364:errorcluster, "VISA resource name out"=w365:refnum<visa-resource-name>)  [unwired: 2 in]
          }
          event "Tilt  X.Motor": Value Change {
            n207 = event-data() -> ("NewVal"=w376:bool)  [unwired: 1 in, 5 out]
            n208 = local read "AxisNumTiltX"() -> (w377:dbl)
            n209 = call <instrlib>:"Enable Disable Motor.vi"("error in (no error)"=w374, "Action (OFF)"=w376, "Axis (1)"=w377, "VISA resource name"=w375) -> ("error out"=w372:errorcluster, "VISA resource name out"=w371:refnum<visa-resource-name>)  [unwired: 2 in]
          }
          event "Tilt  Y.Motor": Value Change {
            n210 = event-data() -> ("NewVal"=w384:bool)  [unwired: 1 in, 5 out]
            n211 = local read "AxisNumTiltY"() -> (w385:dbl)
            n212 = call <instrlib>:"Enable Disable Motor.vi"("error in (no error)"=w382, "Action (OFF)"=w384, "Axis (1)"=w385, "VISA resource name"=w383) -> ("error out"=w378:errorcluster, "VISA resource name out"=w379:refnum<visa-resource-name>)  [unwired: 2 in]
          }
          event "Axis Y.Move": Value Change {
            n213 = event-data() -> ()  [unwired: 1 in, 6 out]
            n214 = flat-sequence {
              frame #0 {
                n215 = Wait (ms)(milliseconds to wait=u32 50) -> ()  [unwired: 1 out]
                n216 = property on="Move Relative" class="DigNum (strict)"("Value"=0) -> ()  [unwired: 2 in, 2 out]
              }
              frame #1 {
                n217 = property on="Move" class="Bool (strict)"("Value"=FALSE) -> ()  [unwired: 2 in, 2 out]
              }
            }
            n218 = property on="Move Relative" class="DigNum (strict)"() -> ("Value"=w389:dbl)  [unwired: 2 in, 2 out]
            n219 = local read "AxisNumY"() -> (w392:dbl)
            n220 = call <instrlib>:"Move Relative.vi"("error in (no error)"=w395, "Position (0 units)"=w389, "Axis (1)"=w392, "VISA resource name"=w396) -> ("error out"=w393:errorcluster, "VISA resource name out"=w394:refnum<visa-resource-name>)  [unwired: 2 in]
            n221 = call <instrlib>:"Read Actual Position.vi"("error in (no error)"=w393, "Axis (1)"=w392, "VISA resource name"=w394) -> ("error out"=w390:errorcluster, "Position (units)"=w388:dbl, "VISA resource name out"=w391:refnum<visa-resource-name>)  [unwired: 2 in]
            n222 = property on="Actual Position" class="DigNum (strict)"("Value"=w388) -> ()  [unwired: 2 in, 2 out]
            n223 = property on="Move Absolute" class="DigNum (strict)"("Value"=w388) -> ()  [unwired: 2 in, 2 out]
          }
          event "Axis Z.Move": Value Change {
            n224 = event-data() -> ()  [unwired: 1 in, 6 out]
            n225 = flat-sequence {
              frame #0 {
                n226 = Wait (ms)(milliseconds to wait=u32 50) -> ()  [unwired: 1 out]
                n227 = property on="Move Relative" class="DigNum (strict)"("Value"=0) -> ()  [unwired: 2 in, 2 out]
              }
              frame #1 {
                n228 = property on="Move" class="Bool (strict)"("Value"=FALSE) -> ()  [unwired: 2 in, 2 out]
              }
            }
            n229 = property on="Move Relative" class="DigNum (strict)"() -> ("Value"=w407:dbl)  [unwired: 2 in, 2 out]
            n230 = local read "AxisNumZ"() -> (w408:dbl)
            n231 = call <instrlib>:"Move Relative.vi"("error in (no error)"=w404, "Position (0 units)"=w407, "Axis (1)"=w408, "VISA resource name"=w405) -> ("error out"=w409:errorcluster, "VISA resource name out"=w410:refnum<visa-resource-name>)  [unwired: 2 in]
            n232 = call <instrlib>:"Read Actual Position.vi"("error in (no error)"=w409, "Axis (1)"=w408, "VISA resource name"=w410) -> ("error out"=w403:errorcluster, "Position (units)"=w406:dbl, "VISA resource name out"=w402:refnum<visa-resource-name>)  [unwired: 2 in]
            n233 = property on="Actual Position" class="DigNum (strict)"("Value"=w406) -> ()  [unwired: 2 in, 2 out]
            n234 = property on="Move Absolute" class="DigNum (strict)"("Value"=w406) -> ()  [unwired: 2 in, 2 out]
          }
          event "Tilt  X.Move": Value Change {
            n235 = event-data() -> ()  [unwired: 1 in, 6 out]
            n236 = flat-sequence {
              frame #0 {
                n237 = Wait (ms)(milliseconds to wait=u32 50) -> ()  [unwired: 1 out]
                n238 = property on="Move Relative" class="DigNum (strict)"("Value"=0) -> ()  [unwired: 2 in, 2 out]
              }
              frame #1 {
                n239 = property on="Move" class="Bool (strict)"("Value"=FALSE) -> ()  [unwired: 2 in, 2 out]
              }
            }
            n240 = local read "AxisNumTiltX"() -> (w422:dbl)
            n241 = property on="Move Relative" class="DigNum (strict)"() -> ("Value"=w421:dbl)  [unwired: 2 in, 2 out]
            n242 = call <instrlib>:"Move Relative.vi"("error in (no error)"=w418, "Position (0 units)"=w421, "Axis (1)"=w422, "VISA resource name"=w419) -> ("error out"=w423:errorcluster, "VISA resource name out"=w424:refnum<visa-resource-name>)  [unwired: 2 in]
            n243 = call <instrlib>:"Read Actual Position.vi"("error in (no error)"=w423, "Axis (1)"=w422, "VISA resource name"=w424) -> ("error out"=w417:errorcluster, "Position (units)"=w420:dbl, "VISA resource name out"=w416:refnum<visa-resource-name>)  [unwired: 2 in]
            n244 = property on="Actual Position" class="DigNum (strict)"("Value"=w420) -> ()  [unwired: 2 in, 2 out]
            n245 = property on="Move Absolute" class="DigNum (strict)"("Value"=w420) -> ()  [unwired: 2 in, 2 out]
          }
          event "Tilt  Y.Move": Value Change {
            n246 = event-data() -> ()  [unwired: 1 in, 6 out]
            n247 = flat-sequence {
              frame #0 {
                n248 = Wait (ms)(milliseconds to wait=u32 50) -> ()  [unwired: 1 out]
                n249 = property on="Move Relative" class="DigNum (strict)"("Value"=0) -> ()  [unwired: 2 in, 2 out]
              }
              frame #1 {
                n250 = property on="Move" class="Bool (strict)"("Value"=FALSE) -> ()  [unwired: 2 in, 2 out]
              }
            }
            n251 = local read "AxisNumTiltY"() -> (w436:dbl)
            n252 = property on="Move Relative" class="DigNum (strict)"() -> ("Value"=w435:dbl)  [unwired: 2 in, 2 out]
            n253 = call <instrlib>:"Move Relative.vi"("error in (no error)"=w432, "Position (0 units)"=w435, "Axis (1)"=w436, "VISA resource name"=w433) -> ("error out"=w437:errorcluster, "VISA resource name out"=w438:refnum<visa-resource-name>)  [unwired: 2 in]
            n254 = call <instrlib>:"Read Actual Position.vi"("error in (no error)"=w437, "Axis (1)"=w436, "VISA resource name"=w438) -> ("error out"=w431:errorcluster, "Position (units)"=w434:dbl, "VISA resource name out"=w430:refnum<visa-resource-name>)  [unwired: 2 in]
            n255 = property on="Actual Position" class="DigNum (strict)"("Value"=w434) -> ()  [unwired: 2 in, 2 out]
            n256 = property on="Move Absolute" class="DigNum (strict)"("Value"=w434) -> ()  [unwired: 2 in, 2 out]
          }
          event "Tilt  X.Abort": Value Change {
            n257 = event-data() -> ()  [unwired: 1 in, 6 out]
            n258 = flat-sequence {
              frame #0 {
                n259 = Wait (ms)(milliseconds to wait=u32 50) -> ()  [unwired: 1 out]
              }
              frame #1 {
                n260 = property on="Abort" class="Bool (strict)"("Value"=FALSE) -> ()  [unwired: 2 in, 2 out]
              }
            }
            n261 = local read "AxisNumTiltX"() -> (w445:dbl)
            n262 = call <instrlib>:"Stop Motion.vi"("error in (no error)"=w450, "Axis (1)"=w445, "VISA resource name"=w451) -> ("error out"=w448:errorcluster, "VISA resource name out"=w449:refnum<visa-resource-name>)  [unwired: 3 in]
            n263 = call <instrlib>:"Read absolute position.vi"("error in (no error)"=w448, "Axis (1)"=w445, "VISA resource name"=w449) -> ("error out"=w446:errorcluster, "Position (units)"=w444:dbl, "VISA resource name out"=w447:refnum<visa-resource-name>)  [unwired: 2 in]
            n264 = property on="Actual Position" class="DigNum (strict)"("Value"=w444) -> ()  [unwired: 2 in, 2 out]
            n265 = property on="Move Absolute" class="DigNum (strict)"("Value"=w444) -> ()  [unwired: 2 in, 2 out]
          }
          event "Tilt  Y.Abort": Value Change {
            n266 = event-data() -> ()  [unwired: 1 in, 6 out]
            n267 = flat-sequence {
              frame #0 {
                n268 = Wait (ms)(milliseconds to wait=u32 50) -> ()  [unwired: 1 out]
              }
              frame #1 {
                n269 = property on="Abort" class="Bool (strict)"("Value"=FALSE) -> ()  [unwired: 2 in, 2 out]
              }
            }
            n270 = local read "AxisNumTiltY"() -> (w457:dbl)
            n271 = call <instrlib>:"Stop Motion.vi"("error in (no error)"=w462, "Axis (1)"=w457, "VISA resource name"=w463) -> ("error out"=w460:errorcluster, "VISA resource name out"=w461:refnum<visa-resource-name>)  [unwired: 3 in]
            n272 = call <instrlib>:"Read absolute position.vi"("error in (no error)"=w460, "Axis (1)"=w457, "VISA resource name"=w461) -> ("error out"=w458:errorcluster, "Position (units)"=w456:dbl, "VISA resource name out"=w459:refnum<visa-resource-name>)  [unwired: 2 in]
            n273 = property on="Move Absolute" class="DigNum (strict)"("Value"=w456) -> ()  [unwired: 2 in, 2 out]
            n274 = property on="Actual Position" class="DigNum (strict)"("Value"=w456) -> ()  [unwired: 2 in, 2 out]
          }
          event "Axis X.Abort": Value Change {
            n275 = event-data() -> ()  [unwired: 1 in, 6 out]
            n276 = flat-sequence {
              frame #0 {
                n277 = Wait (ms)(milliseconds to wait=u32 50) -> ()  [unwired: 1 out]
              }
              frame #1 {
                n278 = property on="Abort" class="Bool (strict)"("Value"=FALSE) -> ()  [unwired: 2 in, 2 out]
              }
            }
            n279 = local read "AxisNumX"() -> (w472:dbl)
            n280 = call <instrlib>:"Stop Motion.vi"("error in (no error)"=w469, "Axis (1)"=w472, "VISA resource name"=w470) -> ("error out"=w473:errorcluster, "VISA resource name out"=w474:refnum<visa-resource-name>)  [unwired: 3 in]
            n281 = call <instrlib>:"Read Actual Position.vi"("error in (no error)"=w473, "Axis (1)"=w472, "VISA resource name"=w474) -> ("error out"=w467:errorcluster, "Position (units)"=w471:dbl, "VISA resource name out"=w468:refnum<visa-resource-name>)  [unwired: 2 in]
            n282 = property on="Actual Position" class="DigNum (strict)"("Value"=w471) -> ()  [unwired: 2 in, 2 out]
            n283 = property on="Move Absolute" class="DigNum (strict)"("Value"=w471) -> ()  [unwired: 2 in, 2 out]
          }
          event "Axis Y.Abort": Value Change {
            n284 = event-data() -> ()  [unwired: 1 in, 6 out]
            n285 = flat-sequence {
              frame #0 {
                n286 = Wait (ms)(milliseconds to wait=u32 50) -> ()  [unwired: 1 out]
              }
              frame #1 {
                n287 = property on="Abort" class="Bool (strict)"("Value"=FALSE) -> ()  [unwired: 2 in, 2 out]
              }
            }
            n288 = local read "AxisNumY"() -> (w484:dbl)
            n289 = call <instrlib>:"Stop Motion.vi"("error in (no error)"=w481, "Axis (1)"=w484, "VISA resource name"=w482) -> ("error out"=w485:errorcluster, "VISA resource name out"=w486:refnum<visa-resource-name>)  [unwired: 3 in]
            n290 = call <instrlib>:"Read absolute position.vi"("error in (no error)"=w485, "Axis (1)"=w484, "VISA resource name"=w486) -> ("error out"=w479:errorcluster, "Position (units)"=w483:dbl, "VISA resource name out"=w480:refnum<visa-resource-name>)  [unwired: 2 in]
            n291 = property on="Actual Position" class="DigNum (strict)"("Value"=w483) -> ()  [unwired: 2 in, 2 out]
            n292 = property on="Move Absolute" class="DigNum (strict)"("Value"=w483) -> ()  [unwired: 2 in, 2 out]
          }
        }
        n293 = Wait (ms)(milliseconds to wait=u32 500) -> ()  [unwired: 1 out]
      }
    }
    frame #3 {
      n294 = call <instrlib>:"Close.vi"("error in (no error)"=w492, "VISA resource name"=w489) -> ()  [unwired: 9 in, 1 out]
      n295 = call <instrlib>:"Close.vi"("error in (no error)"=w490, "VISA resource name"=w491) -> ()  [unwired: 9 in, 1 out]
    }
  }
